vi "获取-已连接路由器SSID.vi"() -> (3 "SSID":string)   [LabVIEW 2013]
panel:
  out "standard output":string caption="标准输出"
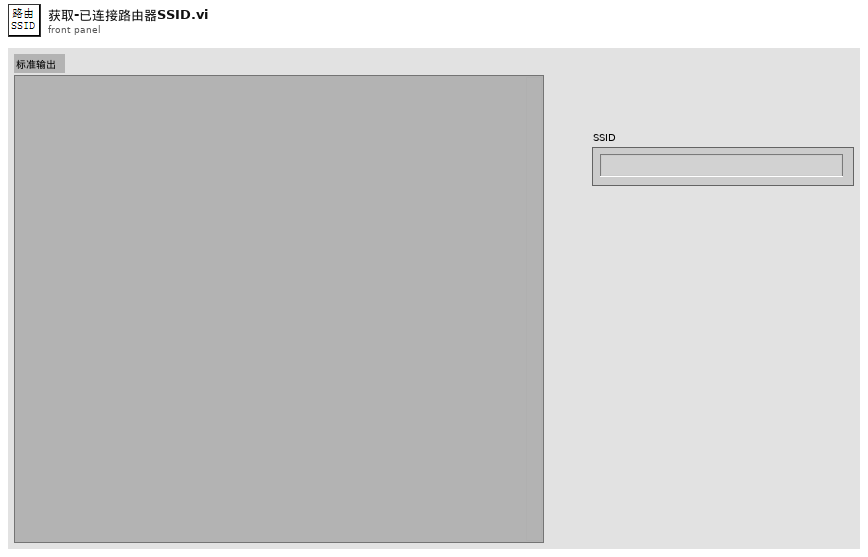
[diagram p1: front panel]
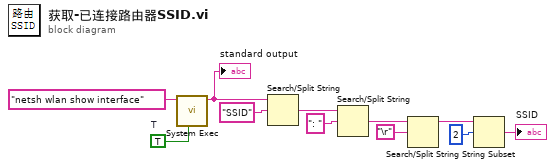
[diagram p0: block diagram]
diagram:
  w10 = TRUE  # T
  n1 = call <vilib>:"System Exec.vi"("run minimized? (F)"=w10, "command line"="netsh wlan show interface") -> ("standard output"=w9:string)  [unwired: 6 in, 3 out]
  "standard output" <- w9
  n2 = Search/Split String(string=w9, search string/char (-)="SSID" ("搜索字符串/字符(-)")) -> (match + rest of string=w7:string)  [unwired: 1 in, 2 out]
  n3 = Search/Split String(string=w7, search string/char (-)=": " ("搜索字符串/字符(-)")) -> (match + rest of string=w5:string)  [unwired: 1 in, 2 out]
  n4 = Search/Split String(string=w5, search string/char (-)="\r") -> (substring before match=w3:string)  [unwired: 1 in, 2 out]
  n5 = String Subset(string=w3, offset (0)=2 ("偏移量(0)")) -> (substring=→"SSID":string)  [unwired: 1 in]
